vi "Run.vi"(8 "error in (no error)":errorcluster caption="entrée d'erreur (pas d'erreur)", 11 "Friedman1.lvclass":refnum<class "Friedman1.lvclass">) -> (0 "error out":errorcluster caption="sortie d'erreur", 2 "Data":T1, 3 "Friedman1.lvclass":refnum<class "Friedman1.lvclass">)   [LabVIEW 2020, in "Friedman1.lvclass"]
doc: "Returns :\n\nX : array of shape [n_samples, n_features]\n The input samples.\n\ny : array of shape [n_samples]\n The output values."
uses:
  Friedman1.lvclass
  Friedman1.lvclass/Friedman1.ctl
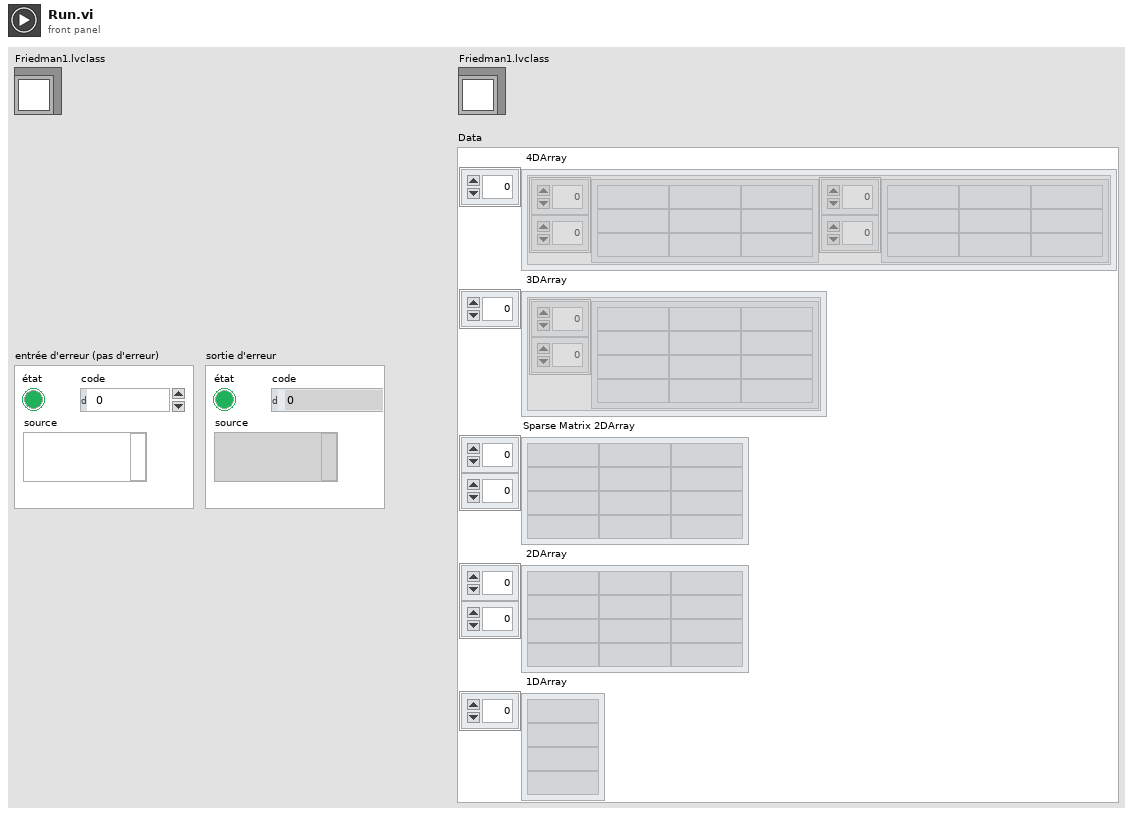
[diagram p1: front panel]
types:
  T1 = cluster{" 4DArray":cluster{"1":string[][], "2":string[][]}[], " 3DArray":cluster{"Tableau":string[][]}[], "Sparse Matrix 2DArray":string[][], " 2DArray":string[][], " 1DArray":string[]}
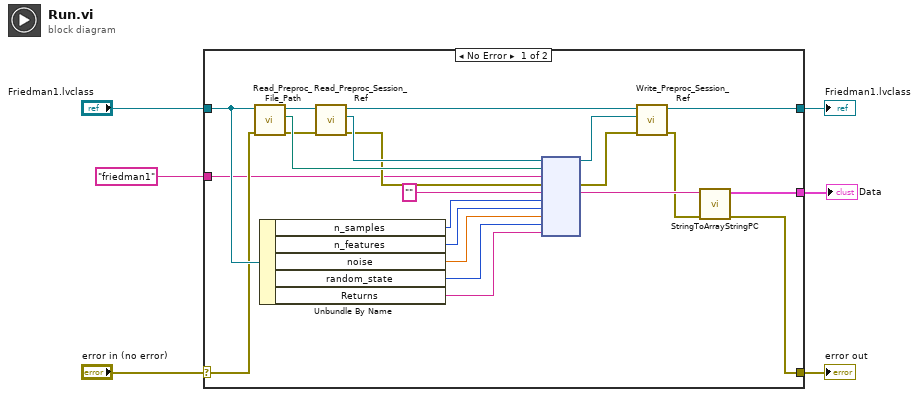
[diagram p0: block diagram]
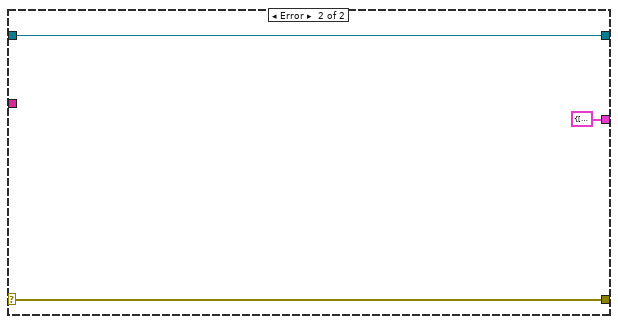
[diagram p2: hidden frame]
diagram:
  n1 = case shown="No Error" "error in (no error)" {
    selector: "error in (no error)" -> [w15 w31]
    tunnel: [w8 w31] -> w5
    tunnel: [w11 w30] -> w3
    tunnel: "Friedman1.lvclass" -> [w16 w30]
    tunnel: "friedman1" -> [w14 _]
    tunnel: [w7 T1 {" 4DArray"=[], " 3DArray"=[], "Sparse Matrix 2DArray"=[], " 2DArray"=[], " 1DArray"=[]} ("Data")] -> w1
    frame No Error {
      n2 = call-dynamic "Read_Preproc_File_Path.vi"("error in (no error)"=w15, "Python in"=w16) -> ("error out"=w23:errorcluster, "File_Path"=w26:path, "Python out"=w28:refnum<class "Friedman1.lvclass">)  [unwired: 7 in]
      n3 = Unbundle By Name(w16) -> ("n_samples"=w19:u32, "n_features"=w18:u32, "noise"=w17:dbl, "random_state"=w13:i32, "Returns"=w12:string)
      n4 = call-dynamic "Read_Preproc_Session_Ref.vi"("error in (no error)"=w23, "Python in"=w28) -> ("error out"=w24:errorcluster, "Session_ref"=w25:refnum<k35>, "Python out"=w27:refnum<class "Friedman1.lvclass">)  [unwired: 7 in]
      n5 = node(w25, w26, w14, w24, "", w19, w18, w17, w13, w12) -> (w20:refnum<k35>, w22:errorcluster, w10:string)  [unwired: 5 in, 2 out]
      n6 = call-dynamic "Write_Preproc_Session_Ref.vi"("error in (no error)"=w22, "Session_ref"=w20, "Python in"=w27) -> ("error out"=w9:errorcluster, "Python out"=w11:refnum<class "Friedman1.lvclass">)  [unwired: 7 in]
      n7 = call "StringToArrayStringPC.vi"("sortie d'erreur"=w9, "Return value"=w10) -> ("sortie d'erreur"=w8:errorcluster, "Data"=w7:T1)  [unwired: 8 in]
    }
    frame Error {
    }
  }
  "error out" <- w5
  "Friedman1.lvclass" <- w3
  "Data" <- w1
